vi "Master Tester.vi"() -> ()   [LabVIEW 2011]
uses:
  Test Info.ctl
  <vilib>/NI Veristand/Execution/Workspace/NI_VS Workspace ExecutionAPI.lvlib
panel:
  out "CurProg":u8(slide) caption="Current configuration progress" scale=0.0..100.0
  out "Total progress":u8(slide) scale=0.0..100.0
  in  "Abort Test":bool
  out "Last attempt (Hz)":dbl
  out "Result":string caption="Last attempt result"
  out "Configuration under test":string
  # "For the included configurations to work without modifications, DAQ Devices are \"Dev1\" \"Dev2\""
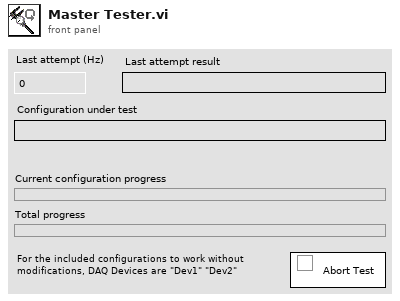
[diagram p1: front panel]
types:
  T1 = typedef "Sysdef Settings.ctl" = cluster{"MaxConv?":bool, "SampleComplete?":bool}
  T2 = typedef "NI_VS Workspace ExecutionAPI.lvlib/WorkspaceAPI.ctl" = refnum<k24>
  T3 = typedef "Test Info.ctl" = cluster{"Last Successful":dbl, "Last Fail":dbl, "Last Try Failed?":bool, "Fail Reasons":bool[]}
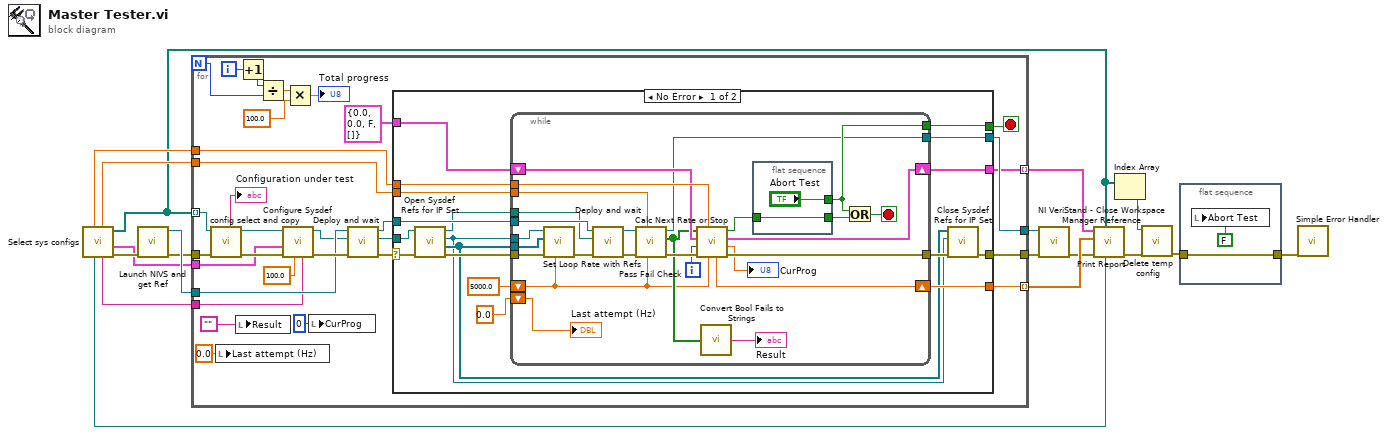
[diagram p0: block diagram]
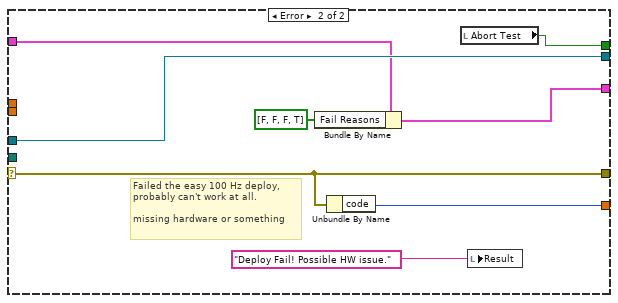
[diagram p2: hidden frame]
diagram:
  n1 = call "Select sys configs.vi"() -> ("error out"=w18:errorcluster, "SysdefSettings"=w1:T1, "paths"=w4:path[], "Target IP Address"=w6:string, "Tolerence (%)"=w17:dbl, "Log file"=w14:path, "Converge target (Hz)"=w16:dbl)  [unwired: 5 in]
  n2 = call "Launch NIVS and get Ref.vi"("error in (no error)"=w18) -> ("error out"=w9:errorcluster, "WorkspaceManager"=w10:T2)  [unwired: 9 in]
  n3 = for {
    N -> [w39]
    tunnel: w4 -> [w48] mode=indexing
    tunnel: w17 -> [w47]
    tunnel: [w30] -> w15 mode=indexing
    tunnel: w16 -> [w46]
    tunnel: w9 -> [w49]
    tunnel: w10 -> [w25]
    tunnel: [w32] -> w13
    tunnel: [w31] -> w11
    tunnel: [w29] -> w8 mode=indexing
    tunnel: w6 -> [w24]
    tunnel: w1 -> [w19]
    i -> [w40]
    stop <- w42 stop-if-true
    n4 = call "config select and copy.vi"("error in (no error)"=w49, "Config in"=w48) -> ("error out"=w33:errorcluster, "UUT Path"=w22:path, "Current Configuration"=→"Configuration under test":string)  [unwired: 7 in]
    n5 = local write "Last attempt (Hz)"(0.0 ("Last attempt (Hz)")) -> ()
    n6 = local write "Result"("") -> ()
    n7 = Increment(x=w40) -> (x+1=w23:i32)
    n8 = Divide(x=w23, y=w39) -> (x/y=w38:dbl)
    n9 = call "Configure Sysdef.vi"("Target IP"=w24, "Target Rate"=100.0, "error in (no error)"=w33, "Set DAQ timing to sample complete?"=w19, "UUT Path"=w22) -> ("error out"=w26:errorcluster, "UUT Path dup"=w21:path)  [unwired: 5 in]
    n10 = Multiply(x=w38, y=100.0) -> (x*y=→"Total progress":dbl)
    n11 = local write "CurProg"(u8 0 ("CurProg")) -> ()
    n12 = call "Deploy and wait.vi"("error in (no error)"=w26, "UUT Path"=w21, "WorkspaceManager in"=w25) -> ("error out"=w44:errorcluster, "UUT Path dup"=w20:path, "WorkspaceManager out"=w45:T2)  [unwired: 6 in]
    n13 = case shown="No Error" w44 {
      selector: w44 -> [w55 w100]
      tunnel: [w56 w100] -> w32
      tunnel: [w67 w103] -> w31
      tunnel: w47 -> [w66 _]
      tunnel: w46 -> [w65 _]
      tunnel: [w64 w99] -> w30
      tunnel: w45 -> [w63 w103]
      tunnel: [w62 w101] -> w42
      tunnel: [w59 w97] -> w29
      tunnel: T3 {"Last Successful"=0.0, "Last Fail"=0.0, "Last Try Failed?"=FALSE, "Fail Reasons"=[]} ("Test Info Out") -> [w58 w98]
      tunnel: w20 -> [w54 _]
      frame No Error {
        n14 = call "Open Sysdef Refs for IP Set.vi"("error in (no error)"=w55, "UUT Path"=w54) -> ("error out"=w53:errorcluster, "Targets"=w52:refnum<k24>[], "SysDef"=w51:refnum<k24>, "UUT Path"=w50:path)  [unwired: 6 in]
        n15 = while {
          shift-right: [w83] -> w64
          shift-left: 0.0 -> [w78]
          tunnel: w63 -> [w93]
          tunnel: [w74] -> w67
          tunnel: w66 -> [w90]
          tunnel: w65 -> [w89]
          shift-right: [w84] -> w59
          shift-left: w58 -> [w85]
          tunnel: [w87] -> w57
          tunnel: [w80] -> w62
          shift-left: 5000.0 -> [w71]
          tunnel: w53 -> [w73]
          tunnel: w51 -> [w70]
          tunnel: w52 -> [w69]
          tunnel: w50 -> [w68]
          i -> [w86]
          stop <- w81 stop-if-true
          n16 = call "Set Loop Rate with Refs.vi"("Target Rate"=w71, "error in (no error)"=w73, "Targets"=w69, "Sysdef"=w70) -> ("error out"=w72:errorcluster)  [unwired: 7 in]
          n17 = call "Deploy and wait.vi"("error in (no error)"=w72, "UUT Path"=w68, "WorkspaceManager in"=w93) -> ("error out"=w92:errorcluster, "WorkspaceManager out"=w91:T2)  [unwired: 6 in, 1 out]
          n18 = call "Pass Fail Check.vi"("Target Rate"=w71, "% tolerance"=w90, "error in (no error)"=w92, "WorkspaceManager in"=w91) -> ("error out"=w88:errorcluster, "Possible Failure Modes"=w82:bool[], "WorkspaceManager out"=w74:T2)  [unwired: 5 in]
          n19 = call "Calc Next Rate or Stop.vi"("Target Rate"=w71, "Converge Target"=w89, "error in (no error)"=w88, "Iteration"=w86, "Test Info In"=w85, "Possible Failure Modes"=w82) -> ("error out"=w87:errorcluster, "CurProg"=→"CurProg":dbl, "Test Info Out"=w84:T3, "Stop?"=w75:bool, "Next Rate"=w83:dbl)  [unwired: 1 in]
          n20 = call "Convert Bool Fails to Strings.vi"("Possible Failure Modes"=w82) -> ("String"=→"Result":string)
          n21 = flat-sequence {
            tunnel: ["Abort Test"] -> w80
            tunnel: [w94] -> w76
            tunnel: w75 -> [w94]
            frame #0 {
            }
          }
          n22 = Or(x=w80, y=w76) -> (x .or. y?=w81:bool)
          "Last attempt (Hz)" <- w78
        }
        n23 = call "Close Sysdef Refs for IP Set.vi"("error in (no error)"=w57, "Sysdef"=w51, "Targets"=w52) -> ("error out"=w56:errorcluster)  [unwired: 8 in]
      }
      frame Error {
        # "Failed the easy 100 Hz deploy,\nprobably can't work at all. \n\nmissing hardware or something"
        n24 = Bundle By Name(cluster=w98, "Fail Reasons"=bool[] [FALSE, FALSE, FALSE, TRUE]) -> (w97:T3)
        n25 = Unbundle By Name(w100) -> ("code"=w99:i32)
        n26 = local read "Abort Test"() -> (w101:bool)
        n27 = local write "Result"("Deploy Fail! Possible HW issue." ("String")) -> ()
      }
    }
  }
  n28 = call <vilib>:"NI VeriStand - Close Workspace Manager Reference.vi"("error in (no error)"=w13, "WorkspaceManager"=w11) -> ("error out"=w12:errorcluster)  [unwired: 9 in]
  n29 = call "Print Report.vi"("Path"=w14, "in4 paths"=w4, "error in (no error)"=w12, "Rates"=w15, "Test Info"=w8) -> ("error out"=w5:errorcluster)  [unwired: 6 in]
  n30 = Index Array(array=w4) -> (element=w3:path)  [unwired: 1 in]
  n31 = call "Delete temp config.vi"("error in (no error)"=w5, "Config in"=w3) -> ("error out"=w2:errorcluster)  [unwired: 9 in]
  n32 = flat-sequence {
    tunnel: [w105] -> w7
    tunnel: w2 -> [w105]
    frame #0 {
      n33 = local write "Abort Test"(FALSE ("Abort Test")) -> ()
    }
  }
  n34 = call <vilib>:"Simple Error Handler.vi"("error in (no error)"=w7) -> ()  [unwired: 4 in, 5 out]
